vi "Fs In Range.vi"(8 "error in (no error)":errorcluster, 10 "Fs":dbl, 11 "Refnum in":refnum<k21>) -> (0 "error out":errorcluster, 2 "coerced(Fs)":dbl, 3 "Refnum out":refnum<k21>)   [LabVIEW 2019, in "Lockin.DAQ.lvclass"]
uses:
  Lockin.DAQ.lvclass
  Typedefs/DAQType-enum.ctl
  <resource>/objmgr/daqmx.rc
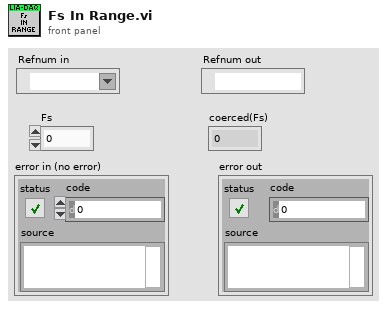
[diagram p1: front panel]
types:
  T1 = typedef "Lockin.DAQ.lvclass/DAQType-enum.ctl" = enum16{"None", "USB 4431", "PXI 446x"}
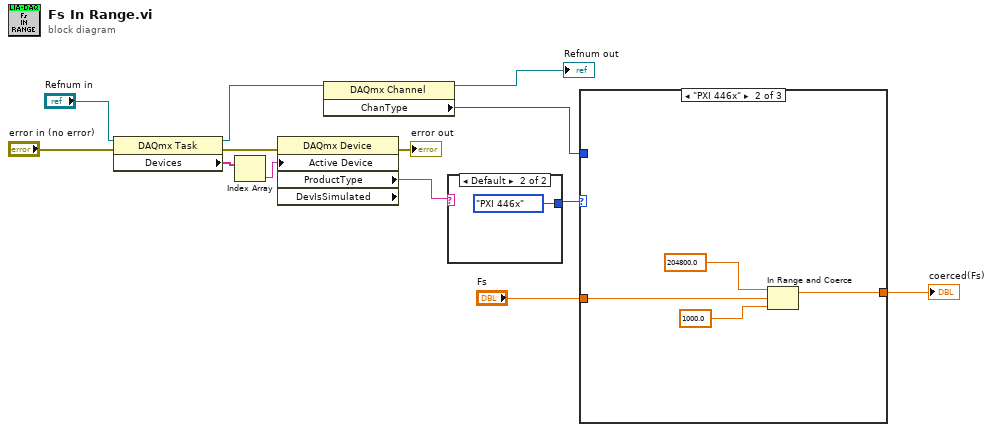
[diagram p0: block diagram]
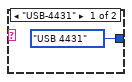
[diagram p2: hidden frame]
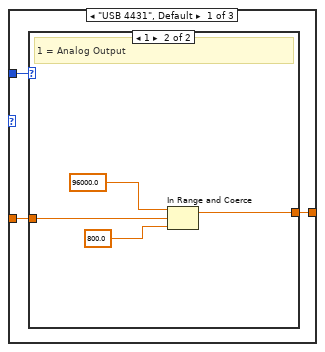
[diagram p3: hidden frame]
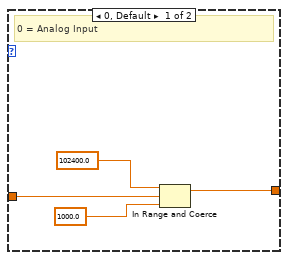
[diagram p4: hidden frame]
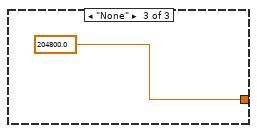
[diagram p5: hidden frame]
diagram:
  n1 = property class="DAQmx Task"(reference="Refnum in", error in="error in (no error)") -> (reference out=w5:refnum<k21>, error out=w13:errorcluster, "Devices"=w12:tag[])
  n2 = Index Array(array=w12) -> (element=w11:tag)  [unwired: 1 in]
  n3 = property class="DAQmx Device" props=["Active Device", "ProductType", "DevIsSimulated"](error in=w13, "Active Device"=w11) -> (error out=→"error out":errorcluster, "ProductType"=w6:string)  [unwired: 1 in, 2 out]
  n4 = property class="DAQmx Channel"(reference=w5) -> (reference out=→"Refnum out":refnum<k21>, "ChanType"=w3:i32)  [unwired: 1 in, 1 out]
  n5 = case shown="Default" w6 {
    tunnel: [DAQType-enum."USB 4431" ("DAQ Type") DAQType-enum."PXI 446x" ("DAQ Type")] -> w9
    frame "USB-4431" {
    }
    frame Default {
    }
  }
  n6 = case shown="\"PXI 446x\"" w9 {
    tunnel: [w18 w27 204800.0 ("upper limit")] -> w1
    tunnel: w3 -> [w17 _ _]
    tunnel: "Fs" -> [w16 w28 _]
    frame "USB 4431", Default {
      n7 = case shown="1" w17 {
        tunnel: [w20 w24] -> w18
        tunnel: w16 -> [w21 w26]
        frame 0, Default {
          # "0 = Analog Input"
          n8 = In Range and Coerce(upper limit=102400.0, x=w21, lower limit=1000.0) -> (coerced(x)=w20:dbl)  [unwired: 1 out]
        }
        frame 1 {
          # "1 = Analog Output"
          n9 = In Range and Coerce(upper limit=96000.0, x=w26, lower limit=800.0) -> (coerced(x)=w24:dbl)  [unwired: 1 out]
        }
      }
    }
    frame "PXI 446x" {
      n10 = In Range and Coerce(upper limit=204800.0, x=w28, lower limit=1000.0) -> (coerced(x)=w27:dbl)  [unwired: 1 out]
    }
    frame "None" {
    }
  }
  "coerced(Fs)" <- w1
